vi "Untitled 1.vi"   [LabVIEW 2014]
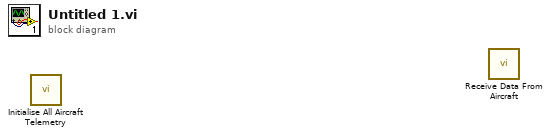
[diagram p0: block diagram]
diagram:
  n1 = call "Initialise All Aircraft Telemetry.vi"() -> ()  [unwired: 11 in, 1 out]
  n2 = call "Receive Data From Aircraft.vi"() -> ()  [unwired: 11 in, 1 out]
